vi "Kill Process by Name.vi"(8 "error in (no error)":errorcluster caption="错误输入（无错误）", 10 "processName":string, 11 "ProcessClass 输入":refnum<class "ProcessClass.lvclass"> caption="DNL_LabVIEW Object in") -> (0 "error out":errorcluster caption="错误输出", 3 "ProcessClass 输出":refnum<class "ProcessClass.lvclass"> caption="DNL_LabVIEW Object out")   [LabVIEW 2012, in "ProcessClass.lvclass"]
uses:
  ProcessClass.lvclass
  ProcessClass.lvclass/ProcessClass.ctl
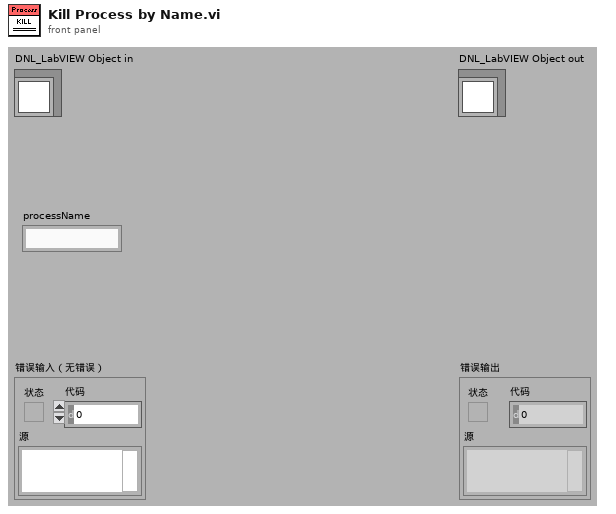
[diagram p1: front panel]
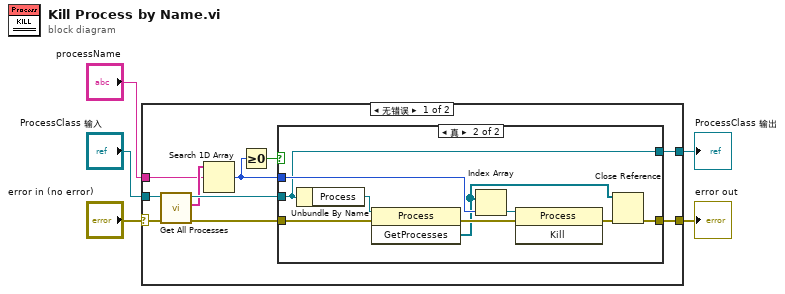
[diagram p0: block diagram]
diagram:
  n1 = case shown="无错误" "error in (no error)" {
    selector: "error in (no error)" -> [w8 w28]
    tunnel: [w6 w28] -> w4
    tunnel: [w9 w27] -> w2
    tunnel: "ProcessClass 输入" -> [w15 w27]
    tunnel: "processName" -> [w12 _]
    frame No Error {
      n2 = call "Get All Processes.vi"("error in (no error)"=w8, "ProcessClass 输入"=w15) -> ("error out"=w7:errorcluster, "Process Names"=w13:string[], "ProcessClass 输出"=w14:refnum<class "ProcessClass.lvclass">)  [unwired: 7 in]
      n3 = Search 1D Array(1D array=w13, element=w12) -> (index of element=w10:i32)  [unwired: 1 in]
      n4 = Greater Or Equal To 0?(x=w10) -> (x >= 0?=w11:bool)
      n5 = case shown="真" w11 {
        tunnel: w14 -> [w17 w24]
        tunnel: w10 -> [_ w25]
        tunnel: [w17 w24] -> w9
        tunnel: w7 -> [w16 w23]
        tunnel: [w16 w19] -> w6
        frame False {
        }
        frame True {
          n6 = Unbundle By Name(w24) -> ("Process"=w26:refnum<k24>)
          n7 = invoke class="Process" method="GetProcesses"(reference=w26, error in=w23) -> (error out=w22:errorcluster, "GetProcesses"=w18:refnum<k24>[])  [unwired: 1 in, 1 out]
          n8 = Index Array(array=w18, index=w25) -> (element=w21:refnum<k24>)
          n9 = invoke class="Process" method="Kill"(reference=w21, error in=w22) -> (error out=w20:errorcluster)  [unwired: 1 in, 2 out]
          n10 = Close Reference(reference=w18, error in (no error)=w20) -> (error out=w19:errorcluster)
        }
      }
    }
    frame Error {
    }
  }
  "error out" <- w4
  "ProcessClass 输出" <- w2
